vi "Count Recursive.vi"(9 "Numbers":i64[](array[numeric]), 10 "Config":u8[](array[numeric]), 11 "Map In":T1(c390)) -> (1 "Count":i64, 3 "Map Out":T1(c390))   [LabVIEW 2021]
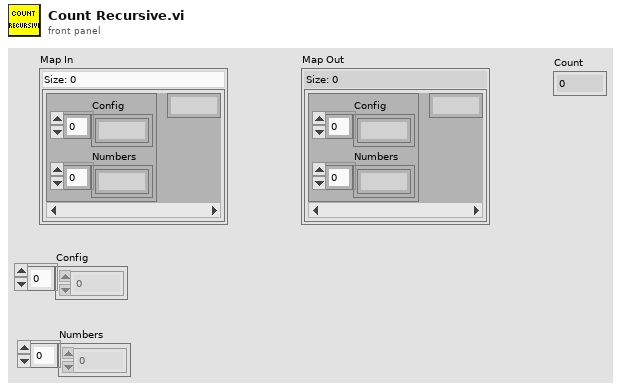
[diagram p1: front panel]
types:
  T1 = map{cluster{"Config":u8[], "Numbers":i64[]}, i64}
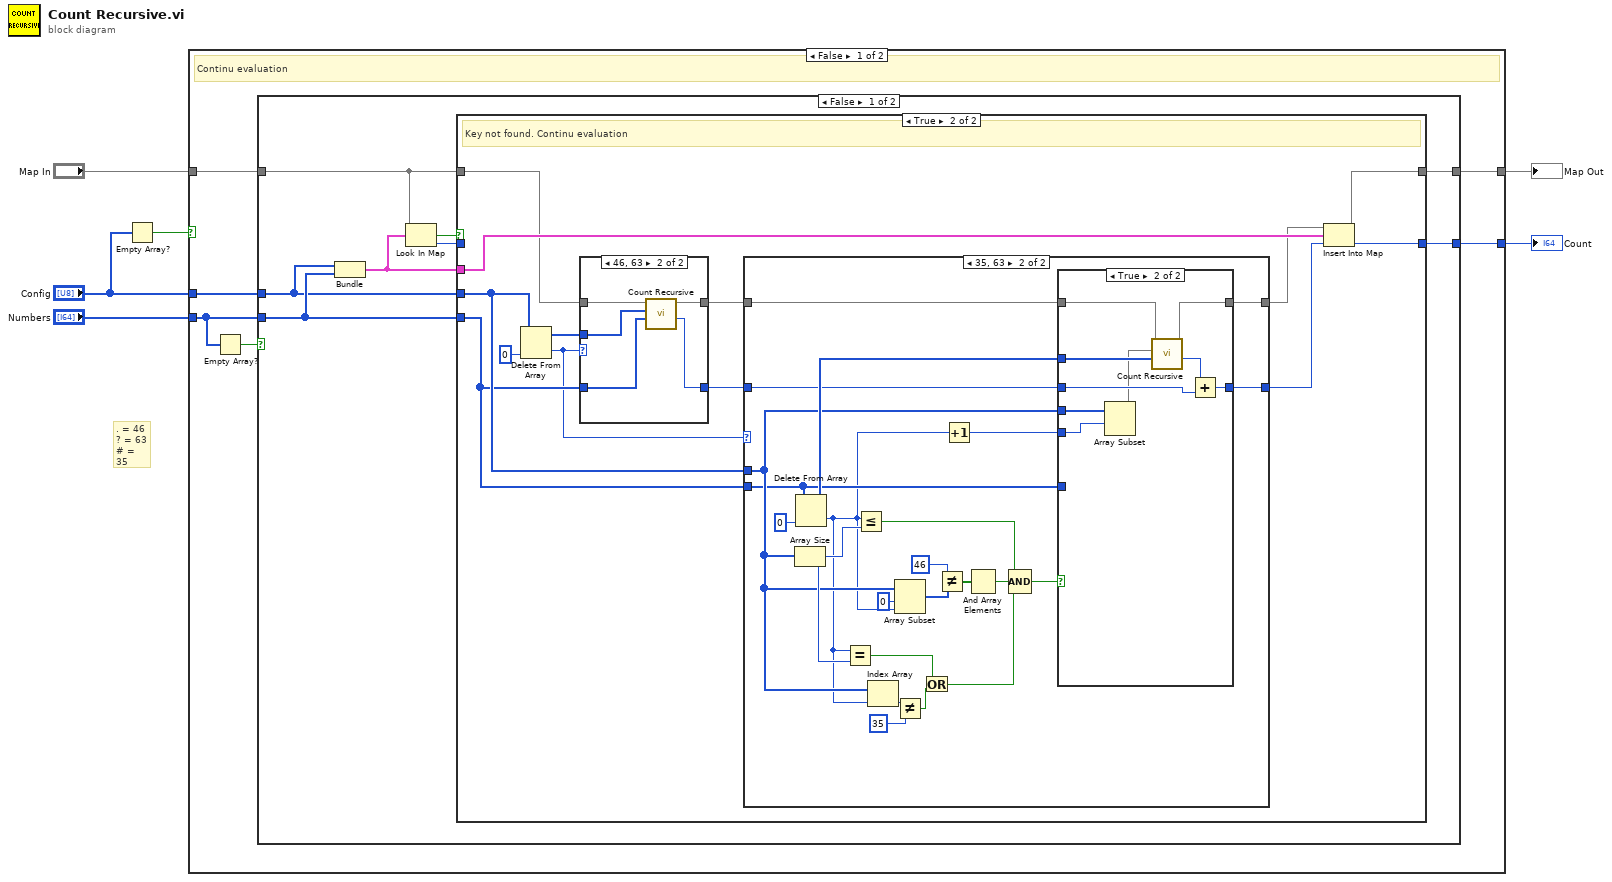
[diagram p0: block diagram]
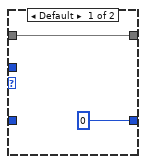
[diagram p5: hidden frame]
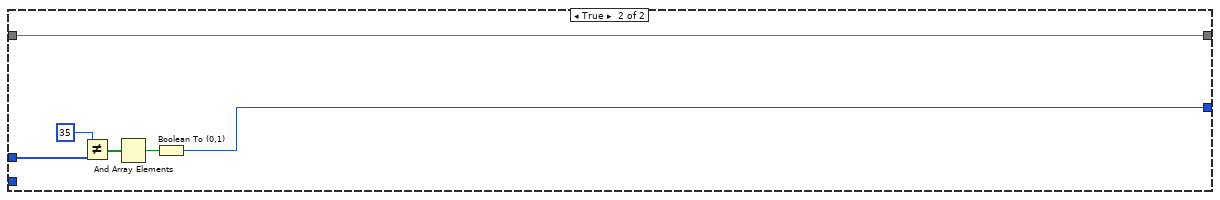
[diagram p6: hidden frame]
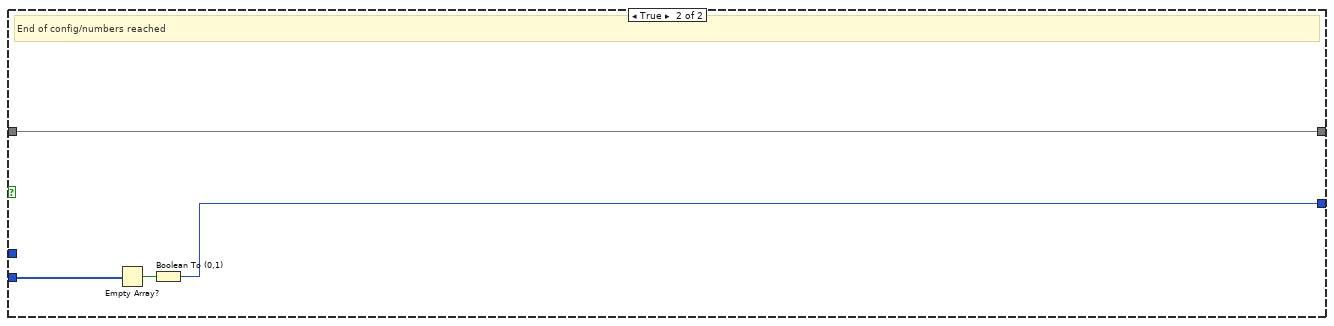
[diagram p7: hidden frame]
diagram:
  # ". = 46\n? = 63\n# = 35"
  n1 = Empty Array?(array="Config") -> (empty?=w1:bool)
  n2 = case shown="False" w1 {
    tunnel: "Map In" -> [w12 w87]
    tunnel: [w10 w87] -> w5
    tunnel: "Config" -> [w9 _]
    tunnel: "Numbers" -> [w8 w86]
    tunnel: [w11 w84] -> w4
    frame False {
      # "Continu evaluation"
      n3 = Empty Array?(array=w8) -> (empty?=w7:bool)
      n4 = case shown="False" w7 {
        tunnel: w12 -> [w20 w78]
        tunnel: [w17 w79] -> w11
        tunnel: [w16 w78] -> w10
        tunnel: w8 -> [w15 _]
        tunnel: w9 -> [w13 w82]
        frame False {
          n5 = Bundle("Config"=w13, "Numbers"=w15) -> (w14:cluster{"Config":u8[], "Numbers":i64[]})  [unwired: 1 in]
          n6 = Look In Map(map=w20, key=w14) -> (key not found?=w19:bool, value=w18:i64)  [unwired: 1 in]
          n7 = case shown="True" w19 {
            tunnel: w20 -> [w21 w31]
            tunnel: w18 -> [w22 _]
            tunnel: [w22 w28] -> w17
            tunnel: [w21 w33] -> w16
            tunnel: w13 -> [_ w25]
            tunnel: w15 -> [_ w24]
            tunnel: w14 -> [_ w34]
            frame False {
              # "Key Found  => Use it"
            }
            frame True {
              # "Key not found. Continu evaluation"
              n8 = Delete From Array(array=w25, index=0) -> (deleted portion=w23:u8, array with subset deleted=w30:u8[])  [unwired: 1 in]
              n9 = case shown="46, 63" w23 {
                tunnel: w31 -> [w71 w77]
                tunnel: [w71 w76] -> w27
                tunnel: w30 -> [_ w74]
                tunnel: w24 -> [_ w75]
                tunnel: [i64 0 ("Count") w73] -> w29
                frame Default {
                }
                frame 46, 63 {
                  n10 = call "Count Recursive.vi"("Numbers"=w75, "Config"=w74, "Map In"=w77) -> ("Count"=w73:i64, "Map Out"=w76:T1)  [unwired: 7 in]
                }
              }
              n11 = case shown="35, 63" w23 {
                tunnel: w29 -> [w36 w55]
                tunnel: [w36 w54] -> w28
                tunnel: w27 -> [w35 w59]
                tunnel: [w35 w56] -> w26
                tunnel: w25 -> [_ w46]
                tunnel: w24 -> [_ w40]
                frame Default {
                }
                frame 35, 63 {
                  n12 = Array Size(array=w46) -> (size(s)=w48:i32)
                  n13 = Delete From Array(array=w40, index=0) -> (deleted portion=w38:i64, array with subset deleted=w57:i64[])  [unwired: 1 in]
                  n14 = Equal?(x=w38, y=w48) -> (x = y?=w47:bool)
                  n15 = Less Or Equal?(x=w38, y=w48) -> (x <= y?=w42:bool)
                  n16 = Index Array(array=w46, index=w38) -> (element=w45:u8)
                  n17 = Array Subset(array=w46, index=0, length=w38) -> (w52:u8[])
                  n18 = Not Equal?(x=w45, y=35) -> (x != y?=w43:bool)
                  n19 = Or(x=w47, y=w43) -> (x .or. y?=w41:bool)
                  n20 = Not Equal?(x=46, y=w52) -> (x != y?=w50:bool[])
                  n21 = Increment(x=w38) -> (x+1=w37:i64)
                  n22 = And Array Elements(Boolean array=w50) -> (logical AND=w49:bool)
                  n23 = Compound Arithmetic op=AND(w42, w49, w41) -> (w53:bool)
                  n24 = case shown="True" w53 {
                    tunnel: w59 -> [w61 w70]
                    tunnel: w57 -> [_ w68]
                    tunnel: [w61 w69] -> w56
                    tunnel: w55 -> [w60 w65]
                    tunnel: [w60 w66] -> w54
                    tunnel: w46 -> [_ w64]
                    tunnel: w37 -> [_ w62]
                    tunnel: w40 -> [_ _]
                    frame False {
                    }
                    frame True {
                      n25 = Array Subset(array=w64, index=w62) -> (w63:u8[])  [unwired: 1 in]
                      n26 = call "Count Recursive.vi"("Numbers"=w68, "Config"=w63, "Map In"=w70) -> ("Count"=w67:i64, "Map Out"=w69:T1)  [unwired: 7 in]
                      n27 = Add(x=w67, y=w65) -> (x+y=w66:i64)
                    }
                  }
                }
              }
              n28 = Insert Into Map(map in=w26, key=w34, value=w28) -> (map out=w33:T1)  [unwired: 2 out]
            }
          }
        }
        frame True {
          n29 = Not Equal?(x=35, y=w82) -> (x != y?=w81:bool[])
          n30 = And Array Elements(Boolean array=w81) -> (logical AND=w80:bool)
          n31 = Boolean To (0,1)(Boolean=w80) -> (0, 1=w79:i16)
        }
      }
    }
    frame True {
      # "End of config/numbers reached"
      n32 = Empty Array?(array=w86) -> (empty?=w85:bool)
      n33 = Boolean To (0,1)(Boolean=w85) -> (0, 1=w84:i16)
    }
  }
  "Map Out" <- w5
  "Count" <- w4
